vi "Mes Remote Table.vi"(5 "mes":T1 {"DateInfo" format="%<%Y/%m/%d>T"}) -> (2 "appended array":string[](array[string]))   [LabVIEW 2014]
uses:
  Type'def/Mes Table.ctl
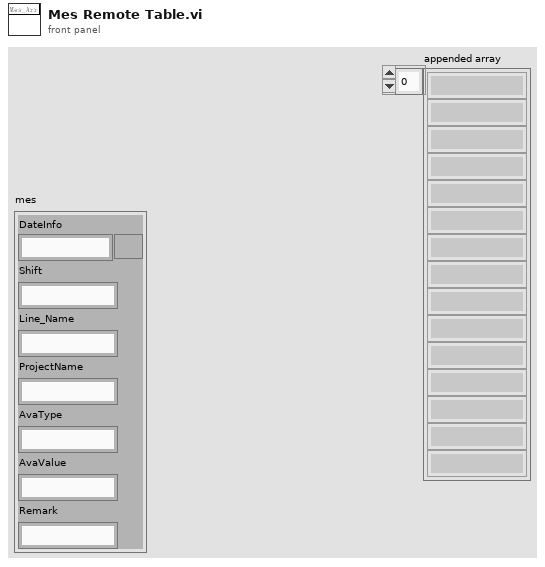
[diagram p1: front panel]
types:
  T1 = typedef "Mes Table.ctl" = cluster{"DateInfo":timestamp, "Shift":string, "Line_Name":string, "ProjectName":string, "AvaType":string, "AvaValue":string, "Remark":string}
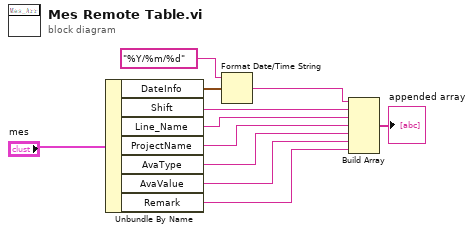
[diagram p0: block diagram]
diagram:
  n1 = Unbundle By Name("mes") -> ("DateInfo"=w10:timestamp, "Shift"=w7:string, "Line_Name"=w6:string, "ProjectName"=w5:string, "AvaType"=w4:string, "AvaValue"=w3:string, "Remark"=w2:string)
  n2 = Format Date/Time String(time format string (%c)="%Y/%m/%d", seconds (now)=w10) -> (date/time string=w8:string)  [unwired: 1 in]
  n3 = Build Array(w8, w7, w6, w5, w4, w3, w2) -> (→"appended array":string[])
